vi "Get response data.vi"(7 "error in":errorcluster, 10 "MES Response":string="<?xml version=\"1.0\" encoding=\"utf-8\"?>\n<soap:Envelope xmlns:xsi=\"http://www.w3.org/2001/XMLSchema-instance\" xmlns:xsd=\"http://www.w3.org/2001/XMLSchema\" xmlns:soap=\"http://schemas.xmlsoap.org/soap/envelope/\">\n  <soap:Body>\n    <ExecuteResponse xmlns=\"http://tempuri.org/\">\n      <ExecuteResult>\n        <Result>string1</Result>\n        <MessageCode>string2</MessageCode>\n        <MessageDescription>string3</MessageDescription>\n        <BoxNo>string4</BoxNo>\n        <PalletNo>string5</PalletNo>\n        <PackingInstruction1>string6</PackingInstruction1>\n        <PackingInstruction2>string7</PackingInstruction2>\n        <PackingInstruction3>string8</PackingInstruction3>\n        <PackingInstruction4>string9</PackingInstruction4>\n        <PackingInstruction5>string10</PackingInstruction5>\n        <SerialCount>int1</SerialCount>\n        <MaxSerialCount>int2</MaxSerialCount>\n        <BoxCount>int3</BoxCount>\n        <MaxBoxCount>int4</MaxBoxCount>\n      </ExecuteResult>\n    </ExecuteResponse>\n  </soap:Body>\n</soap:Envelope>\n") -> (0 "error out":errorcluster, 2 "Parse Errors":string, 3 "Response Data":T1)   [LabVIEW 2023, in "MES.lvlib"]
uses:
  MES.lvlib
  <vilib>/xml/Load XML File.vi
  <vilib>/xml/Close Reference(Node).vi
  <vilib>/xml/Close Reference(NdList).vi
  <resource>/objmgr/DOMUserDefRef.rc
  <vilib>/xml/NI_XML.lvlib
panel:
  out "Array":errorcluster[](array[cluster])
  out "XML File Path":path
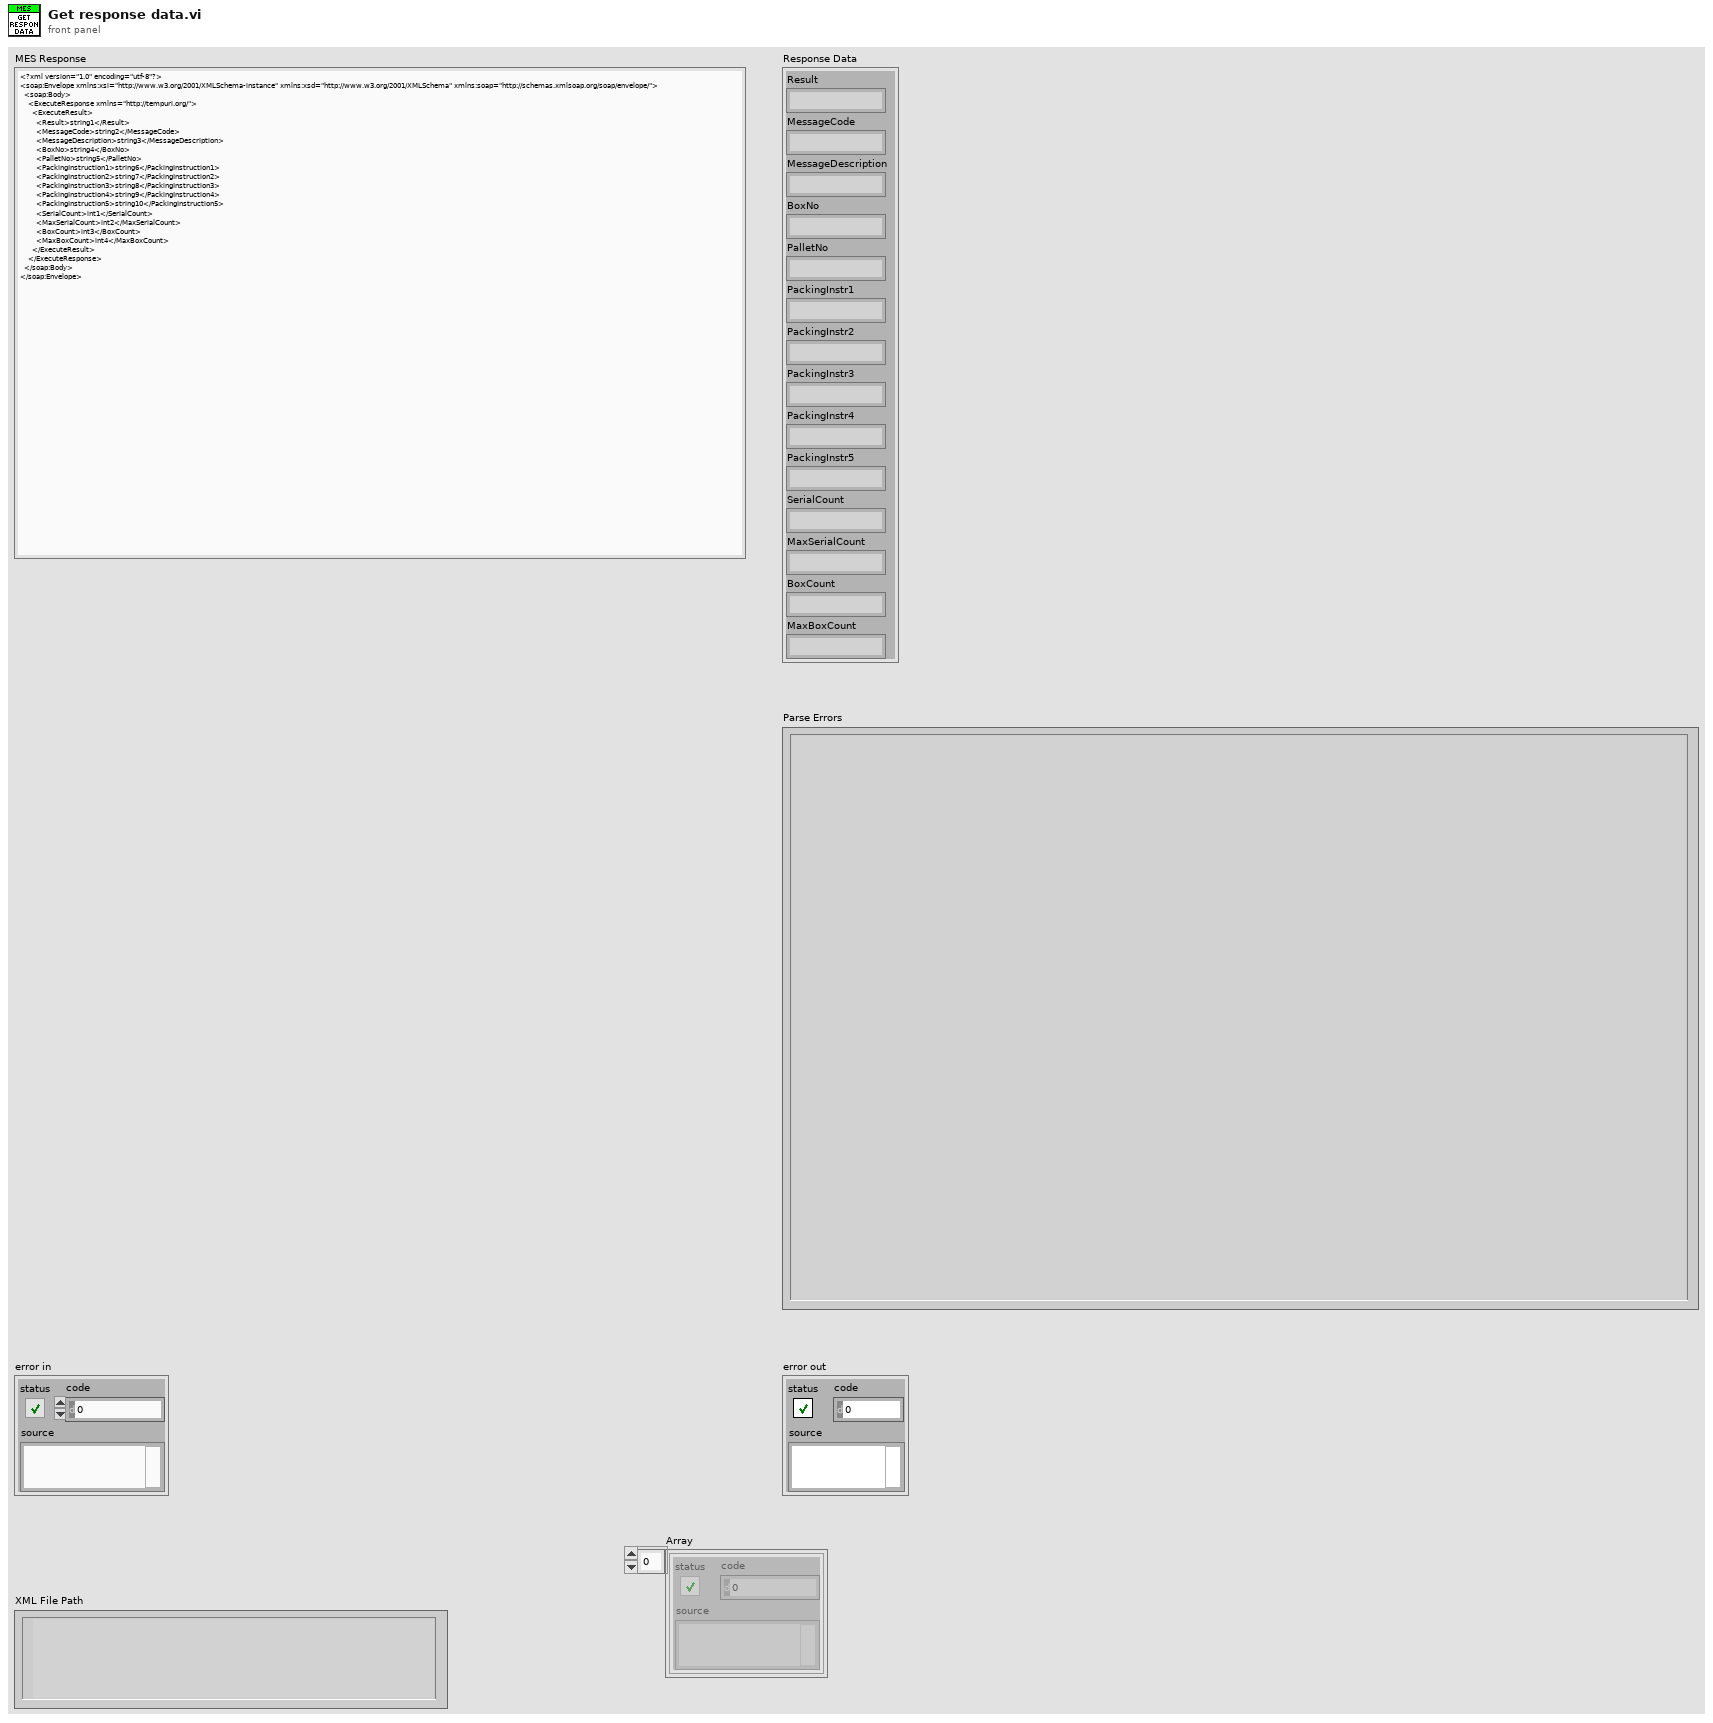
[diagram p1: front panel]
types:
  T1 = cluster{"Result":string, "MessageCode":string, "MessageDescription":string, "BoxNo":string, "PalletNo":string, "PackingInstr1":string, "PackingInstr2":string, "PackingInstr3":string, "PackingInstr4":string, "PackingInstr5":string, "SerialCount":string, "MaxSerialCount":string, "BoxCount":string, "MaxBoxCount":string}
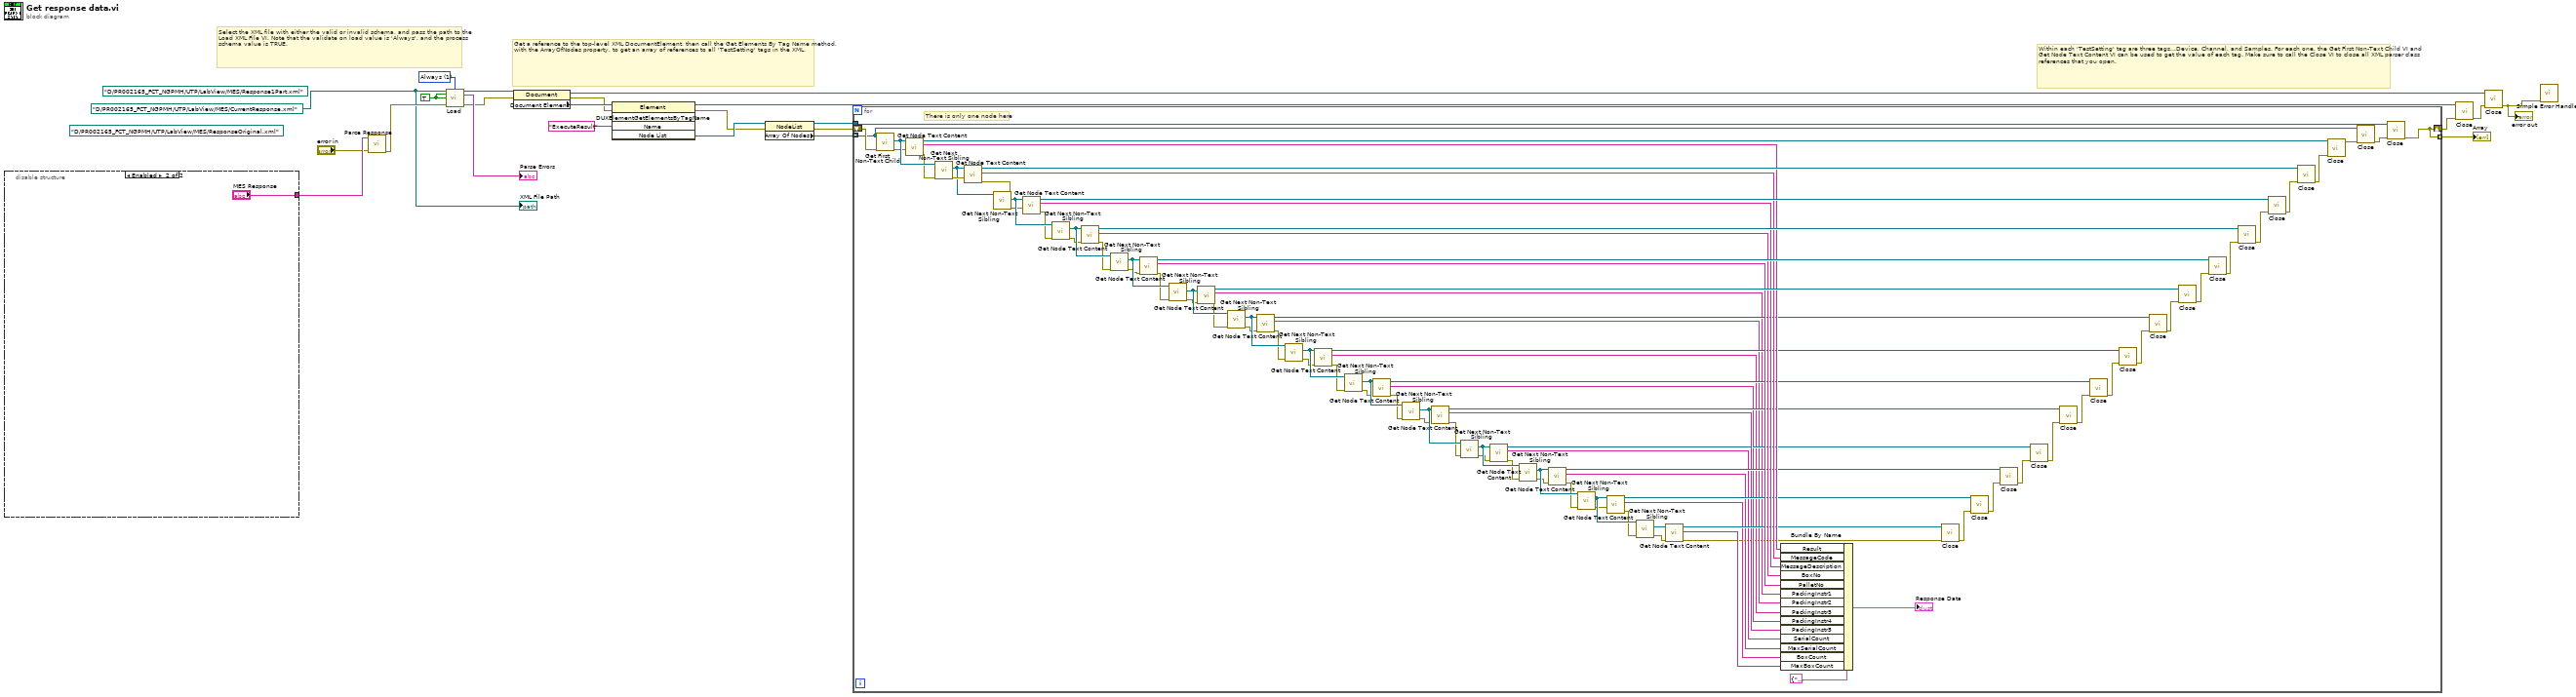
[diagram p0: block diagram]
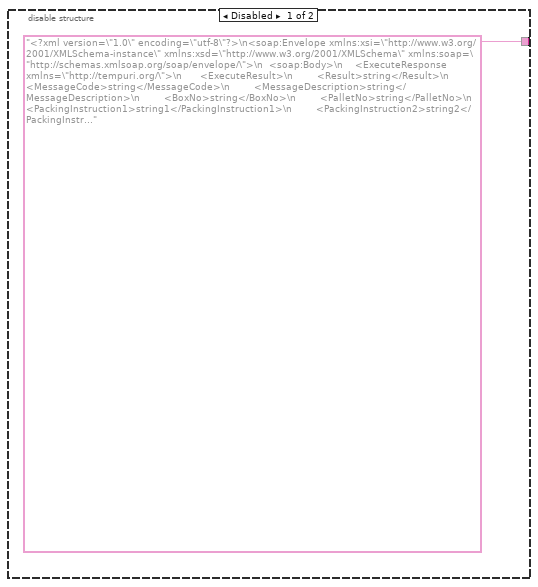
[diagram p2: hidden frame]
diagram:
  w1 = path "D:/PR002165_FCT_NGPMH/UTP/LabView/MES/CurrentResponse.xml" ("file path (use dialog)")
  (unwired) path "D:/PR002165_FCT_NGPMH/UTP/LabView/MES/ResponseOriginal.xml" ("file (use dialog)")
  w23 = 1 items=["Never", "Always", "Auto"] ("Validate On Load")
  w7 = TRUE ("Do Namespaces")
  (unwired) path "D:/PR002165_FCT_NGPMH/UTP/LabView/MES/Response1Part.xml" ("file (use dialog)")
  # "Within each 'TestSetting' tag are three tags...Device, Channel, and Samples. For each one, the Get First Non-Text Child VI and Get Node Text Content VI can be used to get the value of each tag. Make sure to call the Close VI to close all XML parser class references that you open."
  # "Get a reference to the top-level XML DocumentElement, then call the Get Elements By Tag Name method, with the ArrayOfNodes property, to get an array of references to all 'TestSetting' tags in the XML."
  # "Select the XML file with either the valid or invalid schema, and pass the path to the Load XML File VI. Note that the validate on load value is 'Always', and the process schema value is TRUE."
  n1 = disable-structure shown="Enabled" {
    disable-tunnel: ["<?xml version=\"1.0\" encoding=\"utf-8\"?>\n<soap:Envelope xmlns:xsi=\"http://www.w3.org/2001/XMLSchema-instance\" xmlns:xsd=\"http://www.w3.org/2001/XMLSchema\" xmlns:soap=\"http://schemas.xmlsoap.org/soap/envelope/\">\n  <soap:Body>\n    <ExecuteResponse xmlns=\"http://tempuri.org/\">\n      <ExecuteResult>\n        <Result>string</Result>\n        <MessageCode>string</MessageCode>\n        <MessageDescription>string</MessageDescription>\n        <BoxNo>string</BoxNo>\n        <PalletNo>string</PalletNo>\n        <PackingInstruction1>string1</PackingInstruction1>\n        <PackingInstruction2>string2</PackingInstruction2>\n        <PackingInstruction3>string3</PackingInstruction3>\n        <PackingInstruction4>string4</PackingInstruction4>\n        <PackingInstruction5>string</PackingInstruction5>\n        <SerialCount>int</SerialCount>\n        <MaxSerialCount>int</MaxSerialCount>\n        <BoxCount>int</BoxCount>\n        <MaxBoxCount>int</MaxBoxCount>\n      </ExecuteResult>\n    </ExecuteResponse>\n  </soap:Body>\n</soap:Envelope>\n" ("MES Response") "MES Response"] -> w5
    frame Disabled {
    }
    frame Enabled {
    }
  }
  n2 = call "Parce Response.vi"("error in"="error in", "MES Response"=w5) -> ("error out"=w3:errorcluster)  [unwired: 9 in]
  n3 = call-poly <vilib>:"Load.vi"("path to XML document"=w1, "validate on load (Auto)"=w23, "process namespaces (False)"=w7, "process schema (False)"=w7, "error in (no error)"=w3) -> ("DOM document out"=w9:refnum<k20>, "parse errors"=→"Parse Errors":string, "error out"=w8:errorcluster)  [unwired: 2 in, 6 out]
  n4 = property class="Document"(reference=w9, error in=w8) -> (reference out=w10:refnum<k20>, error out=w19:errorcluster, "Document Element"=w20:refnum<k20>)
  n5 = invoke class="Element" method="DUXElementGetElementsByTagName"(reference=w20, error in=w19, "Name"="ExecuteResult" ("Node Name")) -> (reference out=w12:refnum<k20>, error out=w17:errorcluster, "Node List"=w18:refnum<k20>)  [unwired: 2 in, 2 out]
  n6 = property class="NodeList"(reference=w18, error in=w17) -> (reference out=w16:refnum<k20>, error out=w15:errorcluster, "Array Of Nodes"=w14:refnum<k20>[])
  n7 = for {
    tunnel: w14 -> [w91] mode=indexing
    tunnel: w16 -> [w115]
    tunnel: [w114] -> w6 mode=indexing
    shift-right: [w114] -> w13
    shift-left: w15 -> [w92]
    # "There is only one node here"
    n8 = call <vilib>:"Get First Non-Text Child.vi"("error in (no error)"=w92, "node in"=w91) -> ("error out"=w66:errorcluster, "child node"=w113:refnum<k20>)  [unwired: 8 out]
    n9 = call <vilib>:"Get Node Text Content.vi"("error in (no error)"=w66, "node in"=w113) -> ("error out"=w65:errorcluster, "node text"=w94:string, "node out"=w104:refnum<k20>)  [unwired: 7 out]
    n10 = call <vilib>:"Get Next Non-Text Sibling.vi"("error in (no error)"=w65, "node in"=w113) -> ("error out"=w109:errorcluster, "sibling node"=w63:refnum<k20>)  [unwired: 8 out]
    n11 = call <vilib>:"Get Node Text Content.vi"("error in (no error)"=w109, "node in"=w63) -> ("error out"=w64:errorcluster, "node text"=w95:string, "node out"=w105:refnum<k20>)  [unwired: 7 out]
    n12 = call <vilib>:"Get Next Non-Text Sibling.vi"("error in (no error)"=w64, "node in"=w63) -> ("error out"=w49:errorcluster, "sibling node"=w62:refnum<k20>)  [unwired: 8 out]
    n13 = call <vilib>:"Get Node Text Content.vi"("error in (no error)"=w49, "node in"=w62) -> ("error out"=w48:errorcluster, "node text"=w96:string, "node out"=w112:refnum<k20>)  [unwired: 7 out]
    n14 = call <vilib>:"Get Next Non-Text Sibling.vi"("error in (no error)"=w48, "node in"=w62) -> ("error out"=w47:errorcluster, "sibling node"=w61:refnum<k20>)  [unwired: 8 out]
    n15 = call <vilib>:"Get Node Text Content.vi"("error in (no error)"=w47, "node in"=w61) -> ("error out"=w46:errorcluster, "node text"=w97:string, "node out"=w106:refnum<k20>)  [unwired: 7 out]
    n16 = call <vilib>:"Get Next Non-Text Sibling.vi"("error in (no error)"=w46, "node in"=w61) -> ("error out"=w45:errorcluster, "sibling node"=w60:refnum<k20>)  [unwired: 8 out]
    n17 = call <vilib>:"Get Node Text Content.vi"("error in (no error)"=w45, "node in"=w60) -> ("error out"=w44:errorcluster, "node text"=w98:string, "node out"=w107:refnum<k20>)  [unwired: 7 out]
    n18 = call <vilib>:"Get Next Non-Text Sibling.vi"("error in (no error)"=w44, "node in"=w60) -> ("error out"=w43:errorcluster, "sibling node"=w59:refnum<k20>)  [unwired: 8 out]
    n19 = call <vilib>:"Get Node Text Content.vi"("error in (no error)"=w43, "node in"=w59) -> ("error out"=w42:errorcluster, "node text"=w67:string, "node out"=w108:refnum<k20>)  [unwired: 7 out]
    n20 = call <vilib>:"Get Next Non-Text Sibling.vi"("error in (no error)"=w42, "node in"=w59) -> ("error out"=w41:errorcluster, "sibling node"=w58:refnum<k20>)  [unwired: 8 out]
    n21 = call <vilib>:"Get Node Text Content.vi"("error in (no error)"=w41, "node in"=w58) -> ("error out"=w40:errorcluster, "node text"=w68:string, "node out"=w76:refnum<k20>)  [unwired: 7 out]
    n22 = call <vilib>:"Get Next Non-Text Sibling.vi"("error in (no error)"=w40, "node in"=w58) -> ("error out"=w39:errorcluster, "sibling node"=w57:refnum<k20>)  [unwired: 8 out]
    n23 = call <vilib>:"Get Node Text Content.vi"("error in (no error)"=w39, "node in"=w57) -> ("error out"=w38:errorcluster, "node text"=w69:string, "node out"=w77:refnum<k20>)  [unwired: 7 out]
    n24 = call <vilib>:"Get Next Non-Text Sibling.vi"("error in (no error)"=w38, "node in"=w57) -> ("error out"=w37:errorcluster, "sibling node"=w54:refnum<k20>)  [unwired: 8 out]
    n25 = call <vilib>:"Get Node Text Content.vi"("error in (no error)"=w37, "node in"=w54) -> ("error out"=w36:errorcluster, "node text"=w70:string, "node out"=w78:refnum<k20>)  [unwired: 7 out]
    n26 = call <vilib>:"Get Next Non-Text Sibling.vi"("error in (no error)"=w36, "node in"=w54) -> ("error out"=w35:errorcluster, "sibling node"=w53:refnum<k20>)  [unwired: 8 out]
    n27 = call <vilib>:"Get Node Text Content.vi"("error in (no error)"=w35, "node in"=w53) -> ("error out"=w34:errorcluster, "node text"=w81:string, "node out"=w79:refnum<k20>)  [unwired: 7 out]
    n28 = call <vilib>:"Get Next Non-Text Sibling.vi"("error in (no error)"=w34, "node in"=w53) -> ("error out"=w33:errorcluster, "sibling node"=w52:refnum<k20>)  [unwired: 8 out]
    n29 = call <vilib>:"Get Node Text Content.vi"("error in (no error)"=w33, "node in"=w52) -> ("error out"=w32:errorcluster, "node text"=w82:string, "node out"=w80:refnum<k20>)  [unwired: 7 out]
    n30 = call <vilib>:"Get Next Non-Text Sibling.vi"("error in (no error)"=w32, "node in"=w52) -> ("error out"=w31:errorcluster, "sibling node"=w51:refnum<k20>)  [unwired: 8 out]
    n31 = call <vilib>:"Get Node Text Content.vi"("error in (no error)"=w31, "node in"=w51) -> ("error out"=w30:errorcluster, "node text"=w83:string, "node out"=w85:refnum<k20>)  [unwired: 7 out]
    n32 = call <vilib>:"Get Next Non-Text Sibling.vi"("error in (no error)"=w30, "node in"=w51) -> ("error out"=w29:errorcluster, "sibling node"=w50:refnum<k20>)  [unwired: 8 out]
    n33 = call <vilib>:"Get Node Text Content.vi"("error in (no error)"=w29, "node in"=w50) -> ("error out"=w28:errorcluster, "node text"=w84:string, "node out"=w88:refnum<k20>)  [unwired: 7 out]
    n34 = call <vilib>:"Get Next Non-Text Sibling.vi"("error in (no error)"=w28, "node in"=w50) -> ("error out"=w56:errorcluster, "sibling node"=w55:refnum<k20>)  [unwired: 8 out]
    n35 = call <vilib>:"Get Node Text Content.vi"("error in (no error)"=w56, "node in"=w55) -> ("error out"=w27:errorcluster, "node text"=w89:string, "node out"=w90:refnum<k20>)  [unwired: 7 out]
    n36 = Bundle By Name(cluster=T1 {"Result"="", "MessageCode"="", "MessageDescription"="", "BoxNo"="", "PalletNo"="", "PackingInstr1"="", "PackingInstr2"="", "PackingInstr3"="", "PackingInstr4"="", "PackingInstr5"="", "SerialCount"="", "MaxSerialCount"="", "BoxCount"="", "MaxBoxCount"=""}, "Result"=w94, "MessageCode"=w95, "MessageDescription"=w96, "BoxNo"=w97, "PalletNo"=w98, "PackingInstr1"=w67, "PackingInstr2"=w68, "PackingInstr3"=w69, "PackingInstr4"=w70, "PackingInstr5"=w81, "SerialCount"=w82, "MaxSerialCount"=w83, "BoxCount"=w84, "MaxBoxCount"=w89) -> (→"Response Data":T1)
    n37 = call-poly <vilib>:"Close.vi"("error in (no error)"=w27, "node"=w90) -> ("error out"=w87:errorcluster)  [unwired: 7 out]
    n38 = call-poly <vilib>:"Close.vi"("error in (no error)"=w87, "node"=w88) -> ("error out"=w86:errorcluster)  [unwired: 7 out]
    n39 = call-poly <vilib>:"Close.vi"("error in (no error)"=w86, "node"=w85) -> ("error out"=w75:errorcluster)  [unwired: 7 out]
    n40 = call-poly <vilib>:"Close.vi"("error in (no error)"=w75, "node"=w80) -> ("error out"=w74:errorcluster)  [unwired: 7 out]
    n41 = call-poly <vilib>:"Close.vi"("error in (no error)"=w74, "node"=w79) -> ("error out"=w73:errorcluster)  [unwired: 7 out]
    n42 = call-poly <vilib>:"Close.vi"("error in (no error)"=w73, "node"=w78) -> ("error out"=w72:errorcluster)  [unwired: 7 out]
    n43 = call-poly <vilib>:"Close.vi"("error in (no error)"=w72, "node"=w77) -> ("error out"=w71:errorcluster)  [unwired: 7 out]
    n44 = call-poly <vilib>:"Close.vi"("error in (no error)"=w71, "node"=w76) -> ("error out"=w102:errorcluster)  [unwired: 7 out]
    n45 = call-poly <vilib>:"Close.vi"("error in (no error)"=w102, "node"=w108) -> ("error out"=w101:errorcluster)  [unwired: 7 out]
    n46 = call-poly <vilib>:"Close.vi"("error in (no error)"=w101, "node"=w107) -> ("error out"=w100:errorcluster)  [unwired: 7 out]
    n47 = call-poly <vilib>:"Close.vi"("error in (no error)"=w100, "node"=w106) -> ("error out"=w99:errorcluster)  [unwired: 7 out]
    n48 = call-poly <vilib>:"Close.vi"("error in (no error)"=w99, "node"=w112) -> ("error out"=w111:errorcluster)  [unwired: 7 out]
    n49 = call-poly <vilib>:"Close.vi"("error in (no error)"=w111, "node"=w105) -> ("error out"=w116:errorcluster)  [unwired: 7 out]
    n50 = call-poly <vilib>:"Close.vi"("error in (no error)"=w116, "node"=w104) -> ("error out"=w93:errorcluster)  [unwired: 7 out]
    n51 = call-poly <vilib>:"Close.vi"("error in (no error)"=w93, "node"=w91) -> ("error out"=w103:errorcluster)  [unwired: 7 out]
    n52 = call-poly <vilib>:"Close.vi"("error in (no error)"=w103, "node list"=w115) -> ("error out"=w114:errorcluster)  [unwired: 7 out]
  }
  "Array" <- w6
  n53 = call-poly <vilib>:"Close.vi"("error in (no error)"=w13, "node"=w12) -> ("error out"=w11:errorcluster)  [unwired: 7 out]
  n54 = call-poly <vilib>:"Close.vi"("error in (no error)"=w11, "node"=w10) -> ("error out"=w2:errorcluster)  [unwired: 7 out]
  "error out" <- w2
  n55 = call <vilib>:"Simple Error Handler.vi"("error in (no error)"=w2) -> ()  [unwired: 4 in, 5 out]
  "XML File Path" <- w1
